vi "is_setup_ok.vi"(3 "Scan with":refnum<vi>, 4 "Measure with":refnum<vi>, 5 "Array":T1(array[cluster])) -> (0 "Scanner OK":bool, 1 "Acq OK":bool, 2 "All OK":bool)   [LabVIEW 2010]
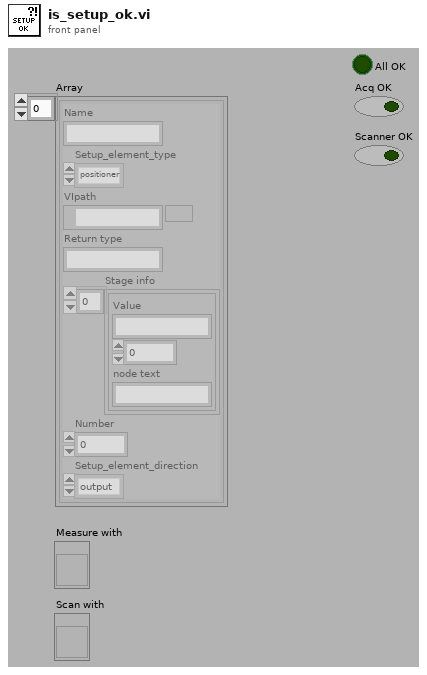
[diagram p1: front panel]
types:
  T1 = cluster{"Name":string, "Setup_element_type":enum16{"positioner", "acquisition", "synchronized"}, "VIpath":path, "Return type":string, "Stage info":cluster{"Value":string, i32, "node text":string}[], "Number":u32, "Setup_element_direction":enum16{"output", "input", "io"}}[]
  T2 = cluster{"Name":string, "Setup_element_type":enum16{"positioner", "acquisition", "synchronized"}, "VIpath":path, "Return type":string, "Stage info":cluster{"Value":string, i32, "node text":string}[], "Number":u32, "Setup_element_direction":enum16{"output", "input", "io"}}
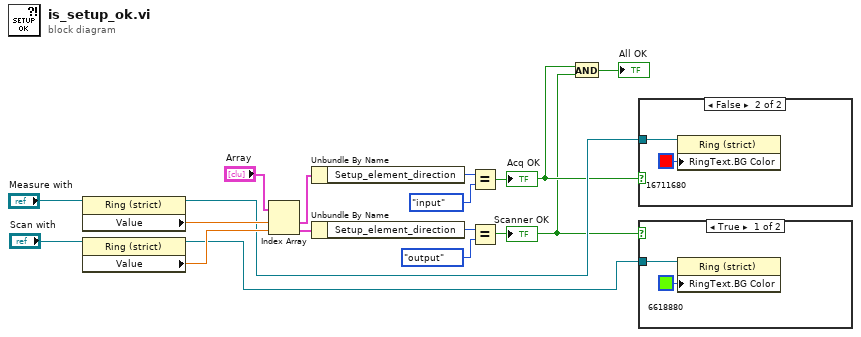
[diagram p0: block diagram]
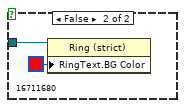
[diagram p2: hidden frame]
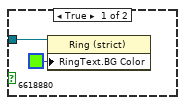
[diagram p3: hidden frame]
diagram:
  n1 = property on="Property Node" class="Ring (strict)"(reference="Measure with") -> (reference out=w7:refnum<vi>, "Value"=w9:dbl)  [unwired: 1 in, 1 out]
  n2 = property on="Property Node" class="Ring (strict)"(reference="Scan with") -> (reference out=w6:refnum<vi>, "Value"=w8:dbl)  [unwired: 1 in, 1 out]
  n3 = Index Array(array="Array", index #1=w9, index #2=w8) -> (element #1=w11:T2, element #2=w12:T2)
  n4 = Unbundle By Name(w11) -> ("Setup_element_direction"=w13:enum16{"output", "input", "io"})
  n5 = Unbundle By Name(w12) -> ("Setup_element_direction"=w15:enum16{"output", "input", "io"})
  n6 = Equal?(x=w13, y=enum16{"output", "input", "io"}."input") -> (x = y?=w5:bool)
  "Acq OK" <- w5
  n7 = Equal?(x=w15, y=enum16{"output", "input", "io"}."output") -> (x = y?=w4:bool)
  "Scanner OK" <- w4
  n8 = And(x=w5, y=w4) -> (x .and. y?=→"All OK":bool)
  n9 = case shown="False" w5 {
    tunnel: w7 -> [w17 w19]
    frame True {
      n10 = property on="Property Node" class="Ring (strict)"(reference=w17, "RingText.BG Color"=u32 6618880) -> ()  [unwired: 1 in, 2 out]
    }
    frame False {
      n11 = property on="Property Node" class="Ring (strict)"(reference=w19, "RingText.BG Color"=u32 16711680) -> ()  [unwired: 1 in, 2 out]
    }
  }
  n12 = case shown="True" w4 {
    tunnel: w6 -> [w21 w23]
    frame True {
      n13 = property on="Property Node" class="Ring (strict)"(reference=w21, "RingText.BG Color"=u32 6618880) -> ()  [unwired: 1 in, 2 out]
    }
    frame False {
      n14 = property on="Property Node" class="Ring (strict)"(reference=w23, "RingText.BG Color"=u32 16711680) -> ()  [unwired: 1 in, 2 out]
    }
  }
